vi "destroyEvents.vi"(8 "error in (no error)":errorcluster, 11 "MonoCommunicator in":refnum<class "MonoCommunicator.lvclass">) -> (0 "error out":errorcluster, 3 "MonoCommunicator out":refnum<class "MonoCommunicator.lvclass">)   [LabVIEW 2016, in "MonoCommunicator.lvclass"]
uses:
  MonoCommunicator.lvclass
  MonoCommunicator.lvclass/MonoCommunicator.ctl
  ts_labview_tcp/TCPCommunicator/TCPCommunicator.lvclass/TCPCommunicator.ctl
  ts_labview_tcp/TCPServer/TCPServer.lvclass
  C:/Users/aanania/Documents/ts_monochromator_windows/ts_labview_tcp/TCPCommunicator/TCPCommunicator.lvclass
  MonoPubSubData/MonoPubSubData.lvclass
  ts_labview_tcp/TCPCommunicator/TCPCommunicator.lvclass
  ts_labview_tcp/TCPComEvents/TCPComEvents.lvclass
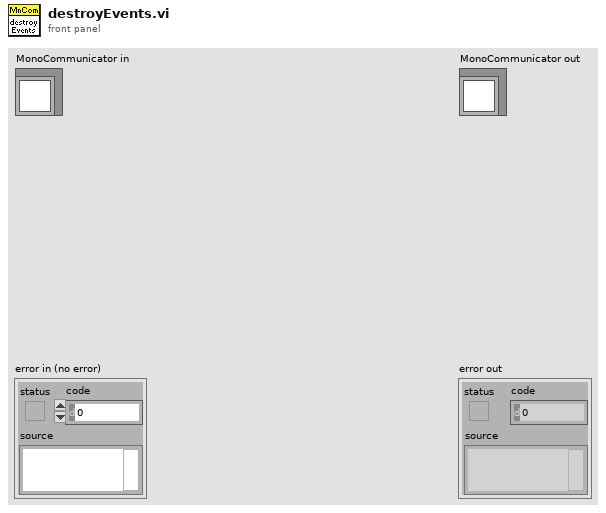
[diagram p1: front panel]
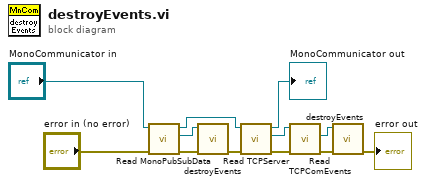
[diagram p0: block diagram]
diagram:
  n1 = call "Read MonoPubSubData.vi"("error in (no error)"="error in (no error)", "MonoCommunicator in"="MonoCommunicator in") -> ("error out"=w9:errorcluster, "MonoPubSubData.lvclass"=w10:refnum<class "MonoPubSubData.lvclass">, "MonoCommunicator out"=w5:refnum<class "MonoCommunicator.lvclass">)  [unwired: 7 in]
  n2 = call "destroyEvents.vi"("error in (no error)"=w9, "MonoPubSubData in"=w10) -> ("error out"=w8:errorcluster)  [unwired: 8 in, 1 out]
  n3 = call "Read TCPServer.vi"("error in (no error)"=w8, "MonoCommunicator in"=w5) -> ("error out"=w7:errorcluster, "TCPServer.lvclass"=w6:refnum<class "TCPServer.lvclass">, "MonoCommunicator out"=→"MonoCommunicator out":refnum<class "MonoCommunicator.lvclass">)  [unwired: 7 in]
  n4 = call "Read TCPComEvents.vi"("error in (no error)"=w7, "TCPCommunicator in"=w6) -> ("error out"=w4:errorcluster, "TCPComEvents.lvclass"=w3:refnum<class "TCPComEvents.lvclass">)  [unwired: 7 in, 1 out]
  n5 = call "destroyEvents.vi"("error in (no error)"=w4, "TCPComEvents in"=w3) -> ("error out"=→"error out":errorcluster)  [unwired: 8 in, 1 out]
